vi "test_contrast_map_filtered_M_stripped.vi"() -> ()   [LabVIEW 2009]
doc: "Copyright (c) 2010 Stepan A. Baranov (stepan@baranov.su)\nAll rights reserved.\nweb-site: www.OCTLab.org"
uses:
  <vilib>/Analysis/NI_AALBase.lvlib
  OCTLib_64.dll
panel:
  out "min":dbl format="%0.2f"
  out "max":dbl format="%0.2f"
  out "version":string
  out "name":string
  out "error out":errorcluster
  out "offset":i32
  out "strip size":i32
  out "A-scan size":i32
  out "# of A-scans":i32
  in  "Small/Big":bool
  out "loop #":i32
  out "RSM_STAT time":u32
  out "LabView time":u32
  out "RSM_STAT Array":dbl[][](array[numeric])
  out "LabView Array":dbl[][](array[numeric])
  in  "stop":bool
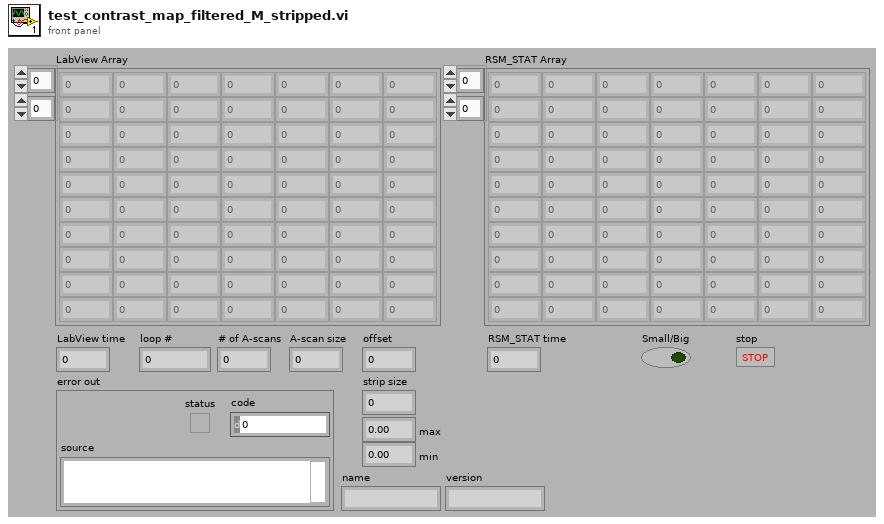
[diagram p1: front panel]
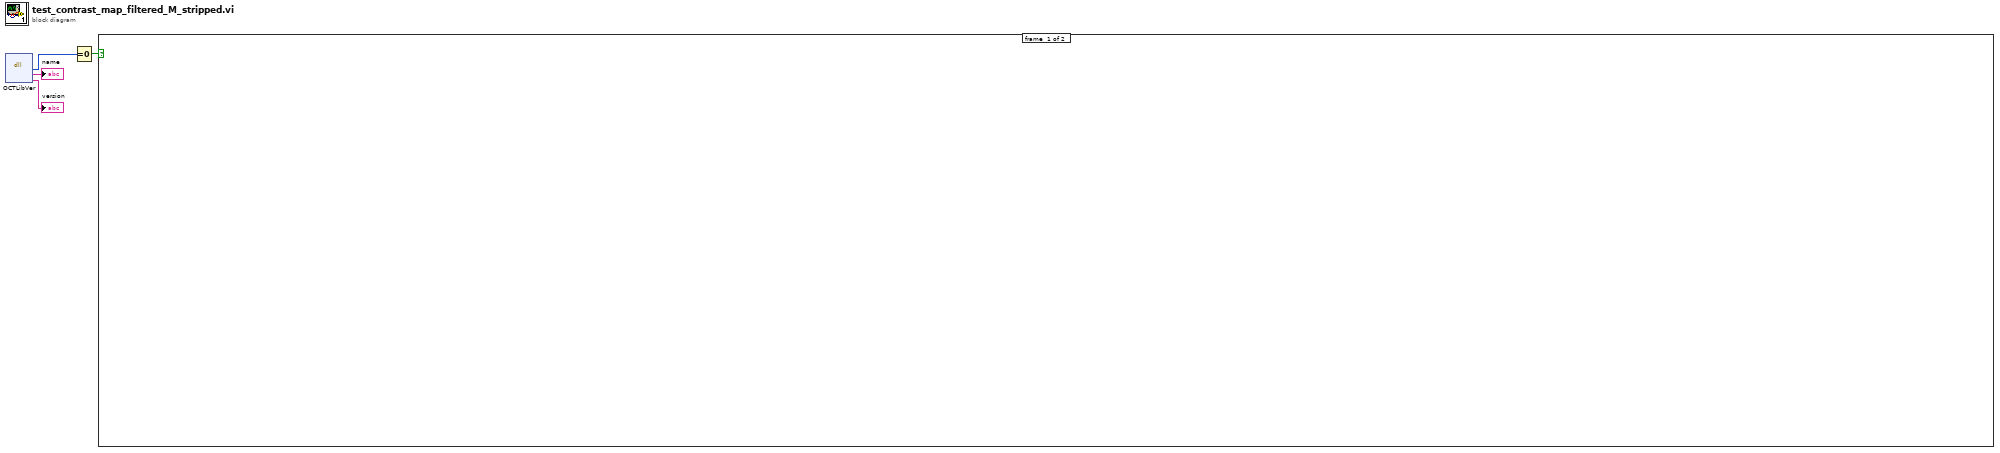
[diagram p0: block diagram]
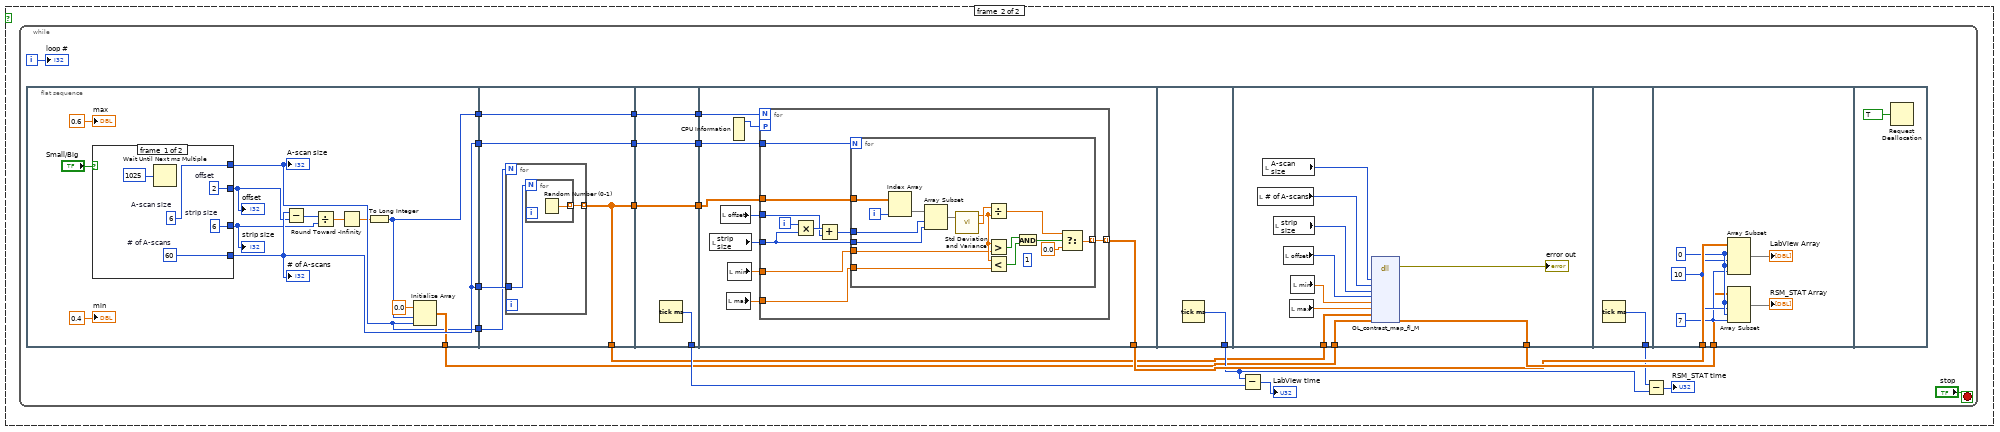
[diagram p2: hidden frame]
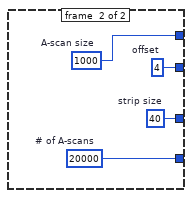
[diagram p3: hidden frame]
diagram:
  n1 = dll-call lib="OCTLib**.*" fn="OCTLibVer"() -> ("status"=w4:i8, "name"=→"name":string, "version"=→"version":string)  [unwired: 5 in, 2 out]
  n2 = Equal To 0?(x=w4) -> (x = 0?=w3:bool)
  n3 = case shown="True" w3 {
    frame #0 {
    }
    frame #1 {
      n4 = while {
        i -> [w17]
        stop <- "stop" stop-if-true
        n5 = flat-sequence {
          tunnel: [w32] -> w13
          tunnel: [w37] -> w12
          tunnel: [w35] -> w11
          tunnel: [w26] -> w6
          tunnel: [w32] -> w5
          tunnel: [w52] -> w16
          tunnel: [w52] -> w14
          tunnel: w13 -> [w51]
          tunnel: w12 -> [w50]
          tunnel: [w48] -> w10
          tunnel: [w49] -> w8
          tunnel: w6 -> [w49]
          tunnel: w5 -> [w48]
          tunnel: [w59] -> w22
          tunnel: [w58] -> w15
          tunnel: w14 -> [w58]
          tunnel: w10 -> [w57]
          tunnel: [w57] -> w9
          tunnel: w8 -> [w56]
          tunnel: [w56] -> w7
          tunnel: [w67] -> w23
          tunnel: w15 -> [w63]
          tunnel: w9 -> [w66]
          tunnel: w7 -> [w65]
          tunnel: [w95] -> w19
          tunnel: w16 -> [w102]
          tunnel: [w105] -> w24
          tunnel: w11 -> [w101]
          tunnel: [w106] -> w20
          tunnel: w24 -> [w107]
          tunnel: w23 -> [w113]
          frame #0 {
            n6 = case shown="False" "Small/Big" {
              tunnel: [w42 w46] -> w37
              tunnel: [w43 w47] -> w32
              tunnel: [w40 w45] -> w29
              tunnel: [w39 w44] -> w31
              frame #0 {
                w39 = 2  # offset
                w40 = 6  # strip size
                w43 = 6  # A-scan size
                w42 = 60  # # of A-scans
                n7 = Wait Until Next ms Multiple(millisecond multiple=u32 1025) -> ()  [unwired: 1 out]
              }
              frame #1 {
                w44 = 4  # offset
                w45 = 40  # strip size
                w47 = 1000  # A-scan size
                w46 = 20000  # # of A-scans
              }
            }
            "# of A-scans" <- w37
            "A-scan size" <- w32
            "strip size" <- w29
            "offset" <- w31
            n8 = Subtract(x=w37, y=w31) -> (x-y=w30:i32)
            n9 = Divide(x=w30, y=w29) -> (x/y=w28:dbl)
            n10 = Round Toward -Infinity(1:w28) -> (0:w27:dbl)
            n11 = To Long Integer(number=w27) -> (32bit integer=w26:i32)
            n12 = Initialize Array(0.0 ("element"), w26, w32) -> (w35:dbl[][])
            "max" <- 0.6 ("min")
            "min" <- 0.4 ("min")
          }
          frame #1 {
            n13 = for {
              N: w50 -> [_]
              tunnel: w51 -> [w54]
              tunnel: [w53] -> w52 mode=indexing
              n14 = for {
                N: w54 -> [_]
                tunnel: [w55] -> w53 mode=indexing
                n15 = Random Number (0-1)() -> (number: 0 to 1=w55:dbl)
              }
            }
          }
          frame #2 {
            n16 = Tick Count (ms)() -> (millisecond timer value=w59:u32)
          }
          frame #3 {
            n17 = local read "strip size"() -> (w60:i32)
            n18 = local read "offset"() -> (w64:i32)
            n19 = local read "max"() -> (w61:dbl)
            n20 = CPU Information() -> (4:w68:i32)  [unwired: 3 out]
            n21 = local read "min"() -> (w62:dbl)
            n22 = for {
              N: w65 -> [_]
              tunnel: [w78] -> w67 mode=indexing
              workers-P: w68 -> [_]
              tunnel: w66 -> [w77]
              tunnel: w60 -> [w72]
              tunnel: w64 -> [w70]
              tunnel: w63 -> [w76]
              tunnel: w62 -> [w75]
              tunnel: w61 -> [w74]
              i -> [w73]
              n23 = Multiply(x=w73, y=w72) -> (x*y=w71:i32)
              n24 = Add(x=w71, y=w70) -> (x+y=w69:i32)
              n25 = for {
                N: w77 -> [_]
                tunnel: w69 -> [w81]
                tunnel: [w88] -> w78 mode=indexing
                tunnel: w72 -> [w80]
                tunnel: w76 -> [w84]
                tunnel: w75 -> [w86]
                tunnel: w74 -> [w85]
                i -> [w83]
                (unwired) 1 ("length")
                n26 = Index Array(array=w84, index (col)=w83) -> (element=w82:dbl[])  [unwired: 1 in]
                n27 = Array Subset(array=w82, index=w81, length=w80) -> (w79:dbl[])
                n28 = call <vilib>:"Std Deviation and Variance.vi"("X"=w79) -> ("mean"=w87:dbl, "standard deviation"=w94:dbl)  [unwired: 1 in, 1 out]
                n29 = Divide(x=w94, y=w87) -> (x/y=w89:dbl)
                n30 = Greater?(x=w87, y=w86) -> (0:w92:bool)
                n31 = Less?(x=w87, y=w85) -> (x < y?=w93:bool)
                n32 = And(x=w92, y=w93) -> (x .and. y?=w91:bool)
                n33 = Select(t=w89, s=w91, f=0.0) -> (s? t:f=w88:dbl)
              }
            }
          }
          frame #4 {
            n34 = Tick Count (ms)() -> (millisecond timer value=w95:u32)
          }
          frame #5 {
            n35 = local read "# of A-scans"() -> (w103:i32)
            n36 = local read "A-scan size"() -> (w104:i32)
            n37 = local read "strip size"() -> (w96:i32)
            n38 = local read "offset"() -> (w97:i32)
            n39 = local read "max"() -> (w98:dbl)
            n40 = local read "min"() -> (w99:dbl)
            n41 = dll-call lib="OCTLib**.*" fn="OL_contrast_map_fl_M"("A-scan size"=w104, "# of A-scan"=w103, "strip size"=w96, "offset"=w97, "min"=w99, "max"=w98, "input"=w102, "data"=w101) -> (error out=→"error out":errorcluster, "data"=w105:dbl[][])  [unwired: 11 in, 1 out]
          }
          frame #6 {
            n42 = Tick Count (ms)() -> (millisecond timer value=w106:u32)
          }
          frame #7 {
            w110 = 10 ("length")
            w109 = 7 ("length")
            w111 = 0 ("index")
            n43 = Array Subset(array=w113, index (row)=w111, length (row)=w110, index (col)=w111, length (col)=w109) -> (→"LabView Array":dbl[][])
            n44 = Array Subset(array=w107, index (row)=w111, length (row)=w110, index (col)=w111, length (col)=w109) -> (→"RSM_STAT Array":dbl[][])
          }
          frame #8 {
            n45 = Request Deallocation(TRUE ("flag")) -> ()
          }
        }
        n46 = Subtract(x=w19, y=w22) -> (x-y=→"LabView time":u32)
        n47 = Subtract(x=w20, y=w19) -> (x-y=→"RSM_STAT time":u32)
        "loop #" <- w17
      }
    }
  }
